vi "CalculateMsgClassPath.vi"(8 "error in (no error)":errorcluster, 10 "Method VI Name":string, 11 "Actor Class Path":path) -> (0 "error out":errorcluster, 3 "Message Class Path":path)   [LabVIEW 2014, in "CS++Actor.lvlib" / "CS++Actor.lvclass"]
doc: "Small helper VI to calculate the new class path of the message."
uses:
  CS++Actor.lvclass
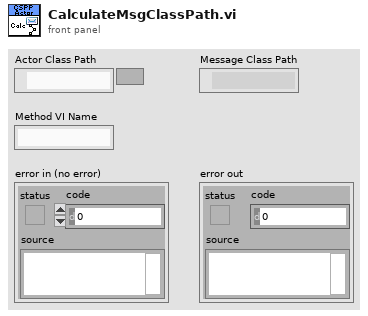
[diagram p1: front panel]
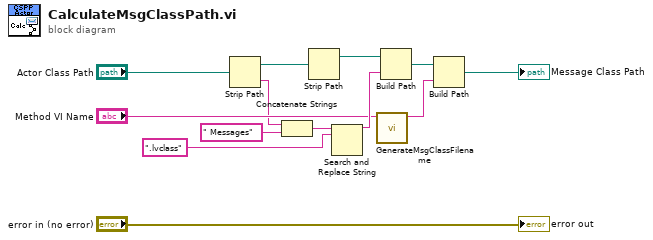
[diagram p0: block diagram]
diagram:
  n1 = Strip Path(path="Actor Class Path") -> (stripped path=w3:path, name=w8:string)
  n2 = Concatenate Strings(w8, " Messages" ("string")) -> (w11:string)
  n3 = Strip Path(path=w3) -> (stripped path=w7:path)  [unwired: 1 out]
  n4 = Search and Replace String(input string=w11, search string=".lvclass" ("string")) -> (result string=w12:string)  [unwired: 6 in, 3 out]
  n5 = call "GenerateMsgClassFilename.vi"("Target Method"="Method VI Name") -> ("Msg Class File Name"=w5:string)  [unwired: 10 in]
  n6 = Build Path(base path=w7, name or relative path=w12) -> (appended path=w6:path)
  n7 = Build Path(base path=w6, name or relative path=w5) -> (appended path=→"Message Class Path":path)
  "error out" <- "error in (no error)"
